vi "CLD 14 CSV file utility.vi"(8 "Error In":errorcluster, 11 "CLD 14 Timer Enum":T1) -> (0 "Error Out":errorcluster, 3 "Array":dbl[](array[numeric]))   [LabVIEW 2009]
doc: "This Utility VI reads from a .csv file."
uses:
  CLD 14 CSV file enum.ctl
  <vilib>/Utility/file.llb/Read From Spreadsheet File (string).vi
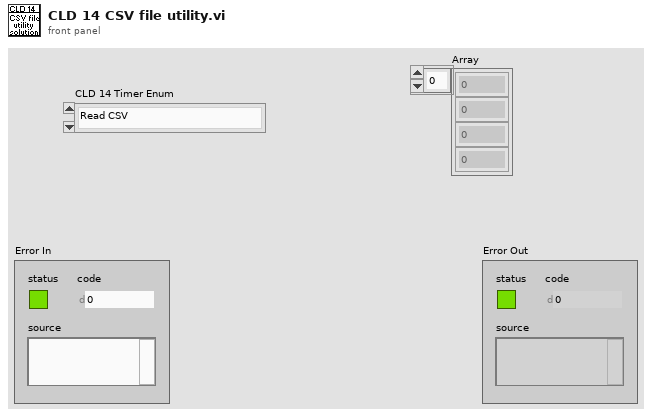
[diagram p1: front panel]
types:
  T1 = typedef "CLD 14 CSV file enum.ctl" = enum16{"Read CSV", "Write CSV"}
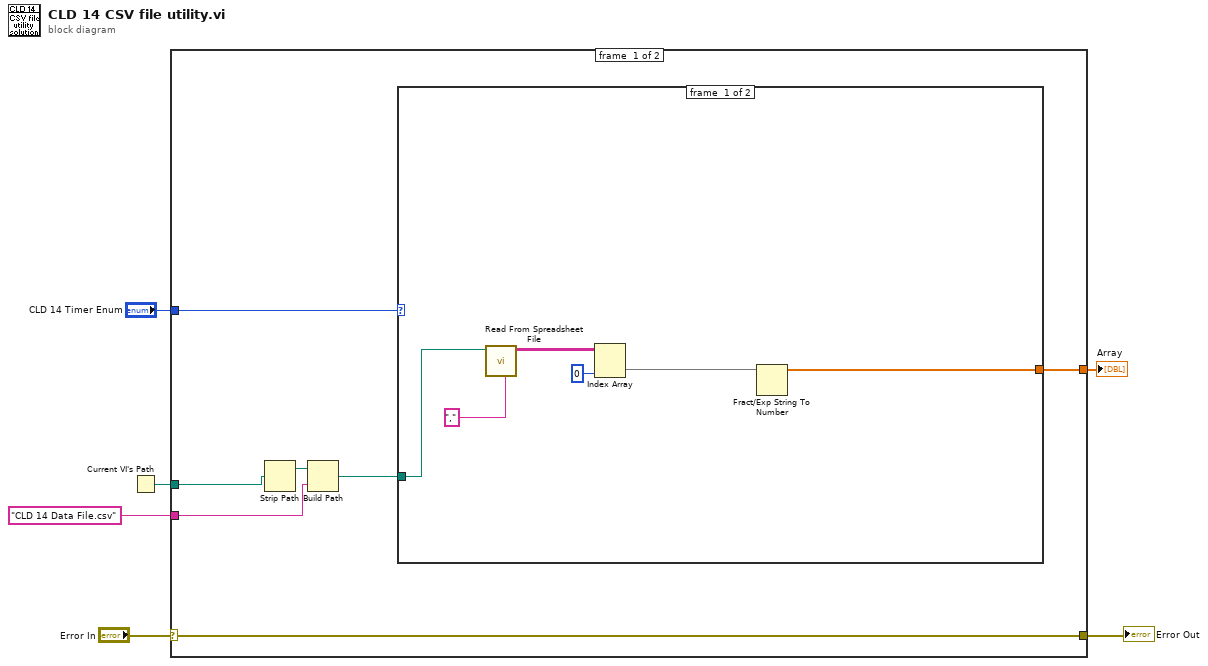
[diagram p0: block diagram]
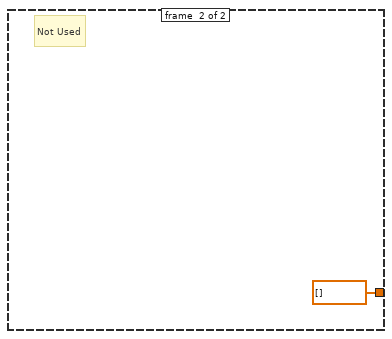
[diagram p2: hidden frame]
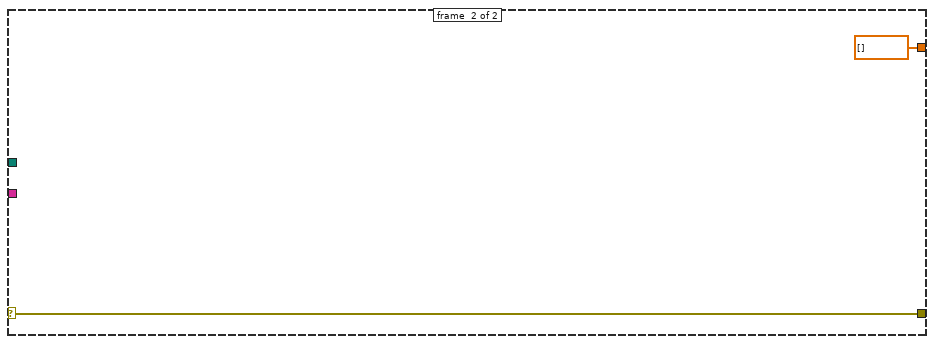
[diagram p3: hidden frame]
diagram:
  n1 = Current VI's Path() -> (path=w5:path)
  n2 = case shown="No Error" "Error In" {
    selector: "Error In" -> [w9 w22]
    tunnel: "CLD 14 Data File.csv" -> [w13 _]
    tunnel: w5 -> [w12 _]
    tunnel: "CLD 14 Timer Enum" -> [w10 _]
    tunnel: [w9 w22] -> w2
    tunnel: [w8 dbl[] []] -> w1
    frame #0 {
      n3 = Strip Path(path=w12) -> (stripped path=w7:path)  [unwired: 1 out]
      n4 = Build Path(base path=w7, name or relative path=w13) -> (appended path=w11:path)
      n5 = case shown="\"Read CSV\", Default" w10 {
        tunnel: w11 -> [w19 _]
        tunnel: [w14 dbl[] []] -> w8
        frame #0 {
          n6 = call-poly <vilib>:"Read From Spreadsheet File.vi"("delimiter (\\t)"="," ("delimiter (\\t)"), "file path (dialog if empty)"=w19) -> ("all rows"=w17:string[][])  [unwired: 5 in, 4 out]
          n7 = Index Array(array=w17, index (col)=0 ("disabled index (col)")) -> (element=w15:string[])  [unwired: 1 in]
          n8 = Fract/Exp String To Number(string=w15) -> (number=w14:dbl[])  [unwired: 3 in, 1 out]
        }
        frame #1 {
          # "Not Used"
        }
      }
    }
    frame #1 {
    }
  }
  "Error Out" <- w2
  "Array" <- w1
